vi "test json edit get or create.vi"(8 "error in (no error)":errorcluster, 11 "Enum":T1(ring)) -> (0 "error out":errorcluster, 1 "JSON out":string, 2 "JSON in":string, 3 "Passed?":bool, 5 "Result":variant)   [LabVIEW 2019, in "labview_json_tests.lvlib"]
uses:
  labview_json_tests.lvlib
  lib/JSON Action.ctl
  854176ce-6913-4507-93ff-74259bbcc79a.vi
  4f657437-8172-4485-bc80-fe3c0f5e02e5.vi
  2eb5ac62-37b8-4a64-bad4-7b844d5cb3ee.vi
  307da32d-3aea-47fb-96ba-a5907bc97348.vi
  17f0fd0c-bcdb-46ee-a433-9aeb7f125615.vi
  96cf0fb6-3c72-4f7d-8904-892807d0a1bb.vi
  59fe4560-8ba1-43eb-ba63-91e62b08ff74.vi
  8ab200a7-ddd1-4c83-9075-6b27156b72a0.vi
  151b51b3-cdff-4f44-b7cf-512c7068f231.vi
  7cf8fa0e-ed30-4591-b618-8510e1b9c6c3.vi
  7fccd278-8607-40f6-9c54-4bdcd723457c.vi
  a2037092-296c-49a0-9406-5a55253d1be9.vi
  64e50d63-3ad6-4fd6-91cf-c341bd7fd43a.vi
  fa781a07-13da-444d-a30b-150b25a8167d.vi
  8b378d6a-7cd8-4d1e-b81a-8e5d845b982b.vi
  e866194e-8ad0-44ef-85b8-025b4f165f38.vi
  ceddfd64-2eb1-41b3-96b1-c2e3a97af537.vi
  42733630-5547-4c55-90bb-661a318f8b3d.vi
  47a0a158-d444-46f2-b9cb-3651ab4d53f4.vi
  e1f56349-deab-4c5b-a68e-11cb9e1278a6.vi
  lib/JSON Edit.vi
  lib/labview_json.lvlib
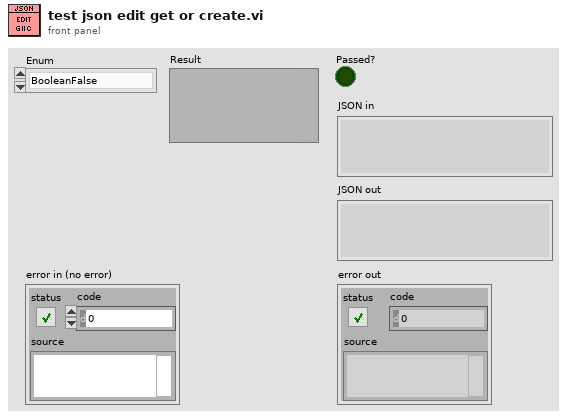
[diagram p1: front panel]
types:
  T1 = enum16{"BooleanFalse", "BooleanTrue", "StringSentence", "StringMultiline", "StringQuoted", "StringEscaped", "IntNumber", "IntMin", "IntMax", "IntI64", "IntI32", "IntI16", "IntI8", "UintNumber", "UintMin", "UintMax", "UintU64", "UintU32", "UintU16", "UintU8", "FloatNumber", "FloatMin", "FloatMax", "FloatZero", "FloatNaN", "FloatExt", "FloatDbl", "FloatSgl", "EnumU32", "EnumU16", "EnumU8", "EnumU32String", "EnumU16String", "EnumU8String", "EnumBadString", "PathAbs", "PathRel", "PathNetwork", "PathFile", "PathEmpty", "PathNaN", "PathCurrentDir", "PathParentDir", "TimeDateTime", "TimeDate", "NullVoid", "NullLVVariant", "NullBoolean", "NullInt", "NullUint", "NullFloat", "NullString", "NullPath", "NullEnum", "NullTime", "NullArray", "NullArrayVoid", "NullArrayLVVariant", "NullObject", "NullObjectVoid", "NullObjectLVVariant", "NullWaveform", "Array1DValues", "Array1DEmpty", "Array1DObject", "Array1DMulti", "Array2DValues", "Array2DEmpty", "Array3DValues", "Array3DEmpty", "ObjectValues", "ObjectEmpty", "ObjectWaveform", "ObjectReorder"}
  T2 = typedef "labview_json.lvlib/JSON Action.ctl" = enum8{"Get or Create", "Get", "Set"}
  T3 = cluster{"I16":i16, "Bool":bool, "String":string, "Array":u32[]}
  T4 = enum16{"Item A", "Item B", "Item C", "Item D", "Item E"}
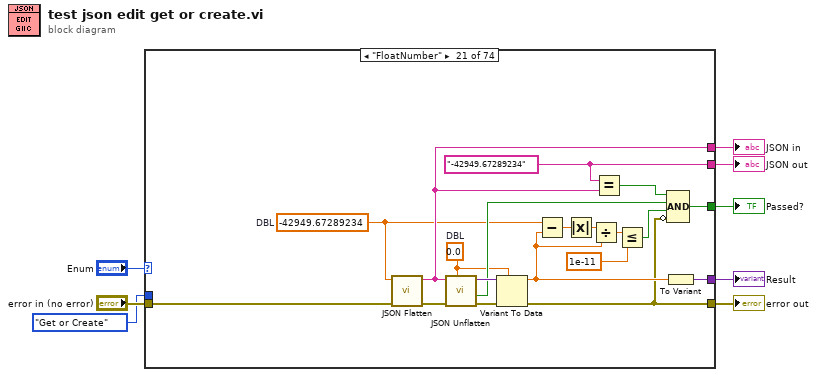
[diagram p0: block diagram]
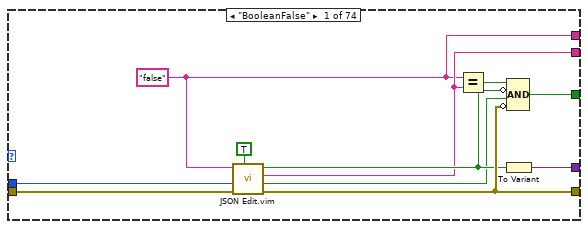
[diagram p2: hidden frame]
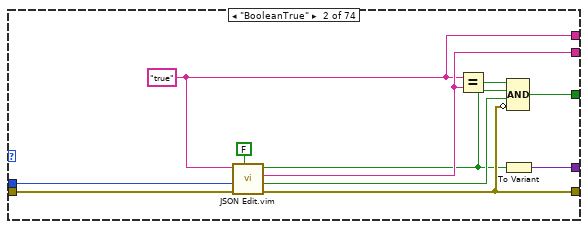
[diagram p3: hidden frame]
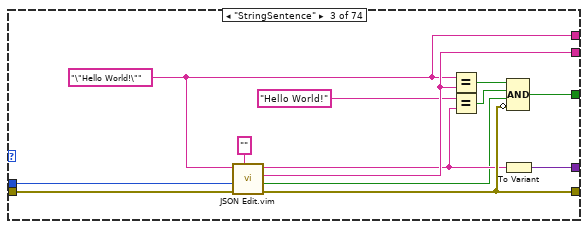
[diagram p4: hidden frame]
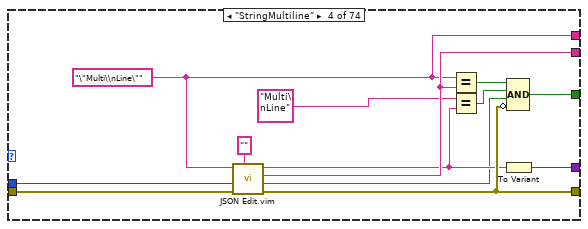
[diagram p5: hidden frame]
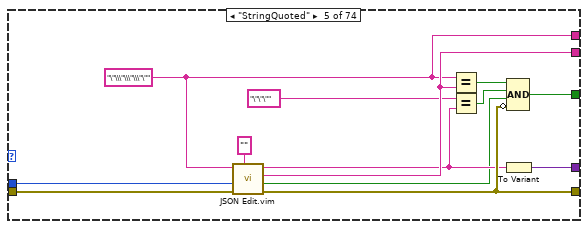
[diagram p6: hidden frame]
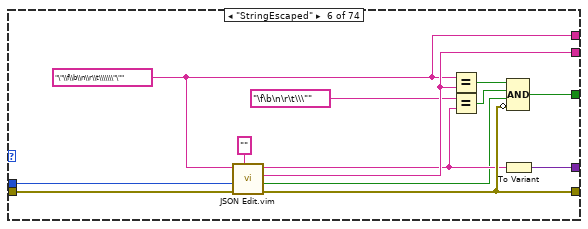
[diagram p7: hidden frame]
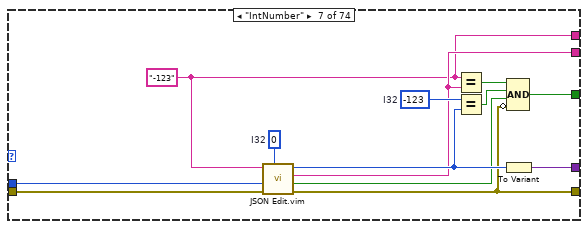
[diagram p8: hidden frame]
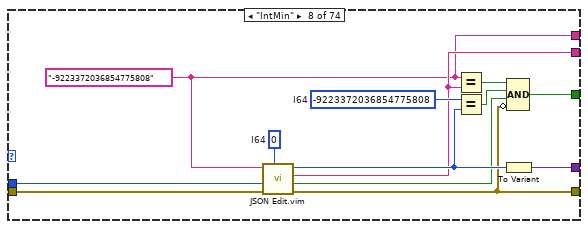
[diagram p9: hidden frame]
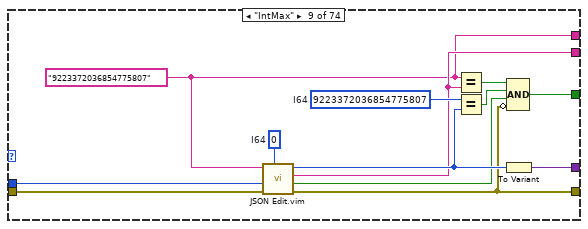
[diagram p10: hidden frame]
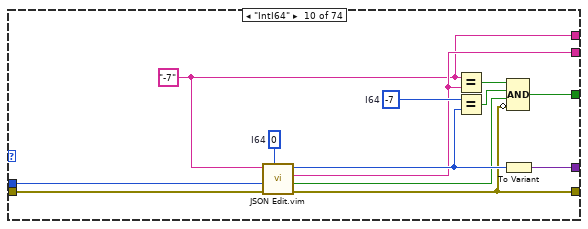
[diagram p11: hidden frame]
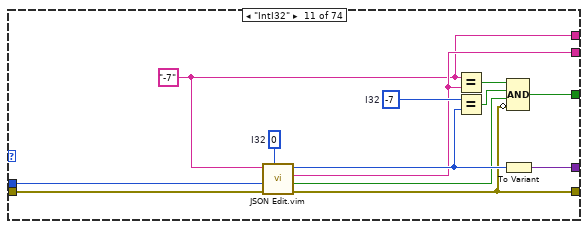
[diagram p12: hidden frame]
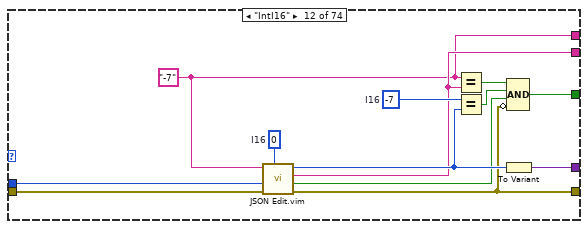
[diagram p13: hidden frame]
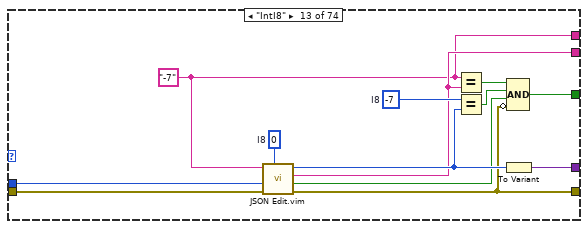
[diagram p14: hidden frame]
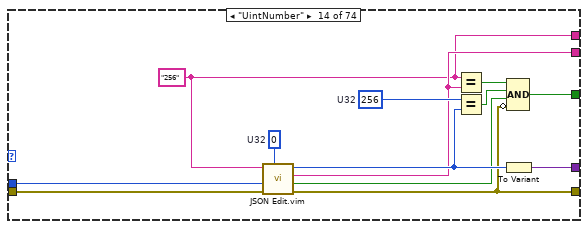
[diagram p15: hidden frame]
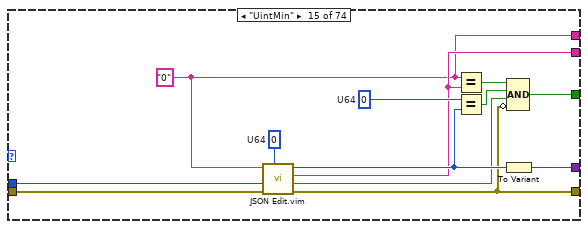
[diagram p16: hidden frame]
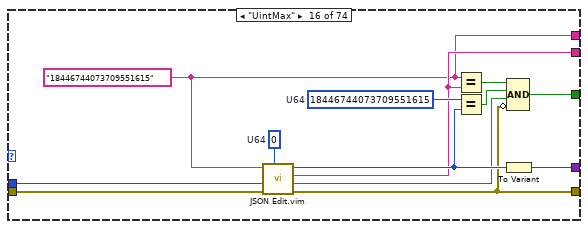
[diagram p17: hidden frame]
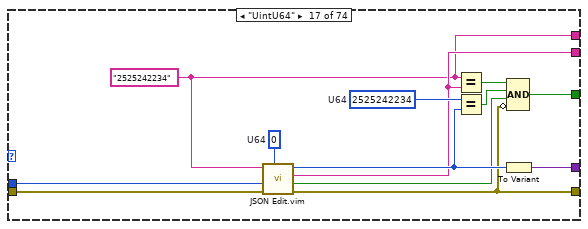
[diagram p18: hidden frame]
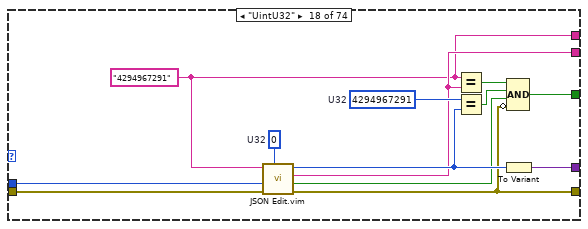
[diagram p19: hidden frame]
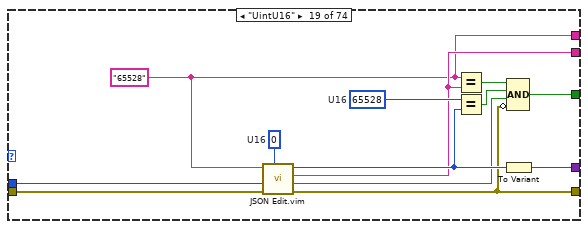
[diagram p20: hidden frame]
diagram:
  n1 = case shown="\"FloatNumber\"" "Enum" {
    tunnel: "error in (no error)" -> [w16 w27 w40 w53 w66 w79 w86 w99 w112 w125 w138 w151 w164 w177 w190 w203 w216 w229 w242 w255 w279 w294 w309 w324 w339 w358 w377 w396 w412 w428 w444 w460 w476 w492 w508 w523 w538 w553 w568 w583 w598 w613 w628 w653 w661 w690 w709 w717 w730 w743 w756 w769 w781 w794 w807 w821 w832 w846 w860 w873 w888 w901 w920 w936 w951 w983 w999 w1015 w1031 w1047 w1064 w1081 w1118 w1138]
    tunnel: [w15 w26 w39 w52 w65 w78 w89 w102 w115 w128 w141 w154 w167 w180 w193 w206 w219 w232 w245 w258 w265 w284 w299 w314 w329 w344 w363 w382 w401 w417 w433 w449 w465 w481 w498 w513 w528 w543 w558 w573 w588 w603 w618 w647 w672 w684 w699 w718 w731 w744 w757 w770 w782 w795 w808 w822 w834 w848 w861 w874 w889 w902 w910 w926 w945 w978 w989 w1005 w1021 w1037 w1058 w1075 w1115 w1132] -> w7
    tunnel: [w18 w29 w42 w55 w68 w81 w94 w107 w120 w133 w146 w159 w172 w185 w198 w211 w224 w237 w250 w263 w282 w297 w312 w327 w342 w361 w380 w399 w415 w431 w447 w463 w479 w495 w511 w526 w541 w556 w571 w586 w601 w616 w631 w656 w678 w693 w712 w723 w736 w749 w762 w775 w787 w800 w813 w827 w839 w853 w866 w879 w894 w907 w923 w939 w954 w986 w1002 w1018 w1034 w1050 w1067 w1084 w1121 w1141] -> w6
    tunnel: [w17 w28 w41 w54 w67 w80 w93 w106 w119 w132 w145 w158 w171 w184 w197 w210 w223 w236 w249 w262 w281 w296 w311 w326 w341 w360 w379 w398 w414 w430 w446 w462 w478 w494 w510 w525 w540 w555 w570 w585 w600 w615 w630 w655 w677 w692 w711 w722 w735 w748 w761 w774 w786 w799 w812 w826 w838 w852 w865 w878 w893 w906 w922 w938 w953 w985 w1001 w1017 w1033 w1049 w1066 w1083 w1120 w1140] -> w5
    tunnel: [w13 w25 w38 w51 w64 w77 w88 w101 w114 w127 w140 w153 w166 w179 w192 w205 w218 w231 w244 w257 w274 w289 w304 w319 w334 w353 w372 w391 w405 w421 w437 w453 w469 w485 w502 w516 w531 w546 w561 w576 w591 w606 w621 w635 w658 w687 w706 w714 w729 w742 w755 w768 w780 w793 w806 w820 w833 w847 w859 w872 w887 w900 w913 w929 w943 w977 w992 w1008 w1024 w1040 w1059 w1076 w1110 w1133] -> w3
    tunnel: [w12 w24 w37 w50 w63 w76 w87 w100 w113 w126 w139 w152 w165 w178 w191 w204 w217 w230 w243 w256 w277 w292 w307 w322 w337 w356 w375 w394 w410 w426 w442 w458 w474 w490 w506 w521 w536 w551 w566 w581 w596 w611 w626 w651 w658 w689 w708 w714 w729 w742 w755 w768 w780 w793 w806 w820 w833 w847 w859 w872 w887 w900 w918 w934 w949 w981 w997 w1013 w1029 w1045 w1062 w1079 w1091 w1136] -> w2
    tunnel: JSON_Action."Get or Create" ("Action (Get or Create)") -> [w10 w22 w36 w49 w62 w75 w83 w96 w109 w122 w135 w148 w161 w174 w187 w200 w213 w226 w239 w252 _ _ _ _ _ _ _ _ _ _ _ _ _ _ _ _ _ _ _ _ _ _ _ _ _ _ _ _ _ _ _ _ _ _ _ _ _ _ _ _ _ _ _ _ _ _ _ _ _ _ _ _ _ _]
    frame "BooleanFalse" {
      w12 = "false" ("JSON in")
      n2 = call "JSON Edit.vim"("Variant in"=TRUE, "error in (no error)"=w16, "Action (Get or Create)"=w10, "JSON in"=w12) -> ("error out"=w15:errorcluster, "Exists?"=w9:bool, "JSON out"=w13:string, "Variant out"=w14:bool)  [unwired: 4 in]
      n3 = Equal?(x=w12, y=w13) -> (x = y?=w19:bool)
      n4 = To Variant(anything=w14) -> (Variant=w17:variant)
      n5 = Compound Arithmetic op=AND(w19, invert w14, w9, invert w15) -> (w18:bool)
    }
    frame "BooleanTrue" {
      w24 = "true" ("JSON in")
      n6 = call "JSON Edit.vim"("Variant in"=FALSE, "error in (no error)"=w27, "Action (Get or Create)"=w22, "JSON in"=w24) -> ("error out"=w26:errorcluster, "Exists?"=w21:bool, "JSON out"=w25:string, "Variant out"=w20:bool)  [unwired: 4 in]
      n7 = Equal?(x=w24, y=w25) -> (x = y?=w30:bool)
      n8 = To Variant(anything=w20) -> (Variant=w28:variant)
      n9 = Compound Arithmetic op=AND(w30, w20, w21, invert w26) -> (w29:bool)
    }
    frame "StringSentence" {
      w37 = "\"Hello World!\"" ("JSON in")
      n10 = call "JSON Edit.vim"("Variant in"="", "error in (no error)"=w40, "Action (Get or Create)"=w36, "JSON in"=w37) -> ("error out"=w39:errorcluster, "Exists?"=w32:bool, "JSON out"=w38:string, "Variant out"=w33:string)  [unwired: 4 in]
      n11 = Equal?(x=w37, y=w38) -> (x = y?=w43:bool)
      n12 = Equal?(x="Hello World!", y=w33) -> (x = y?=w31:bool)
      n13 = To Variant(anything=w33) -> (Variant=w41:variant)
      n14 = Compound Arithmetic op=AND(w43, w31, w32, invert w39) -> (w42:bool)
    }
    frame "StringMultiline" {
      w50 = "\"Multi\\nLine\"" ("JSON in")
      n15 = call "JSON Edit.vim"("Variant in"="", "error in (no error)"=w53, "Action (Get or Create)"=w49, "JSON in"=w50) -> ("error out"=w52:errorcluster, "Exists?"=w45:bool, "JSON out"=w51:string, "Variant out"=w46:string)  [unwired: 4 in]
      n16 = Equal?(x=w50, y=w51) -> (x = y?=w56:bool)
      n17 = Equal?(x="Multi\nLine", y=w46) -> (x = y?=w44:bool)
      n18 = To Variant(anything=w46) -> (Variant=w54:variant)
      n19 = Compound Arithmetic op=AND(w56, w44, w45, invert w52) -> (w55:bool)
    }
    frame "StringQuoted" {
      w63 = "\"\\\"\\\"\\\"\"" ("JSON in")
      n20 = call "JSON Edit.vim"("Variant in"="", "error in (no error)"=w66, "Action (Get or Create)"=w62, "JSON in"=w63) -> ("error out"=w65:errorcluster, "Exists?"=w58:bool, "JSON out"=w64:string, "Variant out"=w59:string)  [unwired: 4 in]
      n21 = Equal?(x=w63, y=w64) -> (x = y?=w69:bool)
      n22 = Equal?(x="\"\"\"", y=w59) -> (x = y?=w57:bool)
      n23 = To Variant(anything=w59) -> (Variant=w67:variant)
      n24 = Compound Arithmetic op=AND(w69, w57, w58, invert w65) -> (w68:bool)
    }
    frame "StringEscaped" {
      w76 = "\"\\f\\b\\n\\r\\t\\\\\\\"\"" ("JSON in")
      n25 = call "JSON Edit.vim"("Variant in"="", "error in (no error)"=w79, "Action (Get or Create)"=w75, "JSON in"=w76) -> ("error out"=w78:errorcluster, "Exists?"=w72:bool, "JSON out"=w77:string, "Variant out"=w73:string)  [unwired: 4 in]
      n26 = Equal?(x=w76, y=w77) -> (x = y?=w82:bool)
      n27 = Equal?(x="\f\b\n\r\t\\\"", y=w73) -> (x = y?=w71:bool)
      n28 = To Variant(anything=w73) -> (Variant=w80:variant)
      n29 = Compound Arithmetic op=AND(w82, w71, w72, invert w78) -> (w81:bool)
    }
    frame "IntNumber" {
      w91 = 0  # I32
      w92 = -123  # I32
      w87 = "-123"
      n30 = call "JSON Edit.vim"("Variant in"=w91, "error in (no error)"=w86, "Action (Get or Create)"=w83, "JSON in"=w87) -> ("error out"=w89:errorcluster, "Exists?"=w85:bool, "JSON out"=w88:string, "Variant out"=w90:i32)  [unwired: 4 in]
      n31 = Equal?(x=w87, y=w88) -> (x = y?=w95:bool)
      n32 = Equal?(x=w92, y=w90) -> (x = y?=w84:bool)
      n33 = To Variant(anything=w90) -> (Variant=w93:variant)
      n34 = Compound Arithmetic op=AND(w95, w84, w85, invert w89) -> (w94:bool)
    }
    frame "IntMin" {
      w104 = i64 0  # I64
      w105 = i64 -9223372036854775808  # I64
      w100 = "-9223372036854775808"
      n35 = call "JSON Edit.vim"("Variant in"=w104, "error in (no error)"=w99, "Action (Get or Create)"=w96, "JSON in"=w100) -> ("error out"=w102:errorcluster, "Exists?"=w98:bool, "JSON out"=w101:string, "Variant out"=w103:i64)  [unwired: 4 in]
      n36 = Equal?(x=w100, y=w101) -> (x = y?=w108:bool)
      n37 = Equal?(x=w105, y=w103) -> (x = y?=w97:bool)
      n38 = To Variant(anything=w103) -> (Variant=w106:variant)
      n39 = Compound Arithmetic op=AND(w108, w97, w98, invert w102) -> (w107:bool)
    }
    frame "IntMax" {
      w117 = i64 0  # I64
      w118 = i64 9223372036854775807  # I64
      w113 = "9223372036854775807"
      n40 = call "JSON Edit.vim"("Variant in"=w117, "error in (no error)"=w112, "Action (Get or Create)"=w109, "JSON in"=w113) -> ("error out"=w115:errorcluster, "Exists?"=w111:bool, "JSON out"=w114:string, "Variant out"=w116:i64)  [unwired: 4 in]
      n41 = Equal?(x=w113, y=w114) -> (x = y?=w121:bool)
      n42 = Equal?(x=w118, y=w116) -> (x = y?=w110:bool)
      n43 = To Variant(anything=w116) -> (Variant=w119:variant)
      n44 = Compound Arithmetic op=AND(w121, w110, w111, invert w115) -> (w120:bool)
    }
    frame "IntI64" {
      w130 = i64 0  # I64
      w131 = i64 -7  # I64
      w126 = "-7"
      n45 = call "JSON Edit.vim"("Variant in"=w130, "error in (no error)"=w125, "Action (Get or Create)"=w122, "JSON in"=w126) -> ("error out"=w128:errorcluster, "Exists?"=w124:bool, "JSON out"=w127:string, "Variant out"=w129:i64)  [unwired: 4 in]
      n46 = Equal?(x=w126, y=w127) -> (x = y?=w134:bool)
      n47 = Equal?(x=w131, y=w129) -> (x = y?=w123:bool)
      n48 = To Variant(anything=w129) -> (Variant=w132:variant)
      n49 = Compound Arithmetic op=AND(w134, w123, w124, invert w128) -> (w133:bool)
    }
    frame "IntI32" {
      w143 = 0  # I32
      w144 = -7  # I32
      w139 = "-7"
      n50 = call "JSON Edit.vim"("Variant in"=w143, "error in (no error)"=w138, "Action (Get or Create)"=w135, "JSON in"=w139) -> ("error out"=w141:errorcluster, "Exists?"=w137:bool, "JSON out"=w140:string, "Variant out"=w142:i32)  [unwired: 4 in]
      n51 = Equal?(x=w139, y=w140) -> (x = y?=w147:bool)
      n52 = Equal?(x=w144, y=w142) -> (x = y?=w136:bool)
      n53 = To Variant(anything=w142) -> (Variant=w145:variant)
      n54 = Compound Arithmetic op=AND(w147, w136, w137, invert w141) -> (w146:bool)
    }
    frame "IntI16" {
      w156 = i16 0  # I16
      w157 = i16 -7  # I16
      w152 = "-7"
      n55 = call "JSON Edit.vim"("Variant in"=w156, "error in (no error)"=w151, "Action (Get or Create)"=w148, "JSON in"=w152) -> ("error out"=w154:errorcluster, "Exists?"=w150:bool, "JSON out"=w153:string, "Variant out"=w155:i16)  [unwired: 4 in]
      n56 = Equal?(x=w152, y=w153) -> (x = y?=w160:bool)
      n57 = Equal?(x=w157, y=w155) -> (x = y?=w149:bool)
      n58 = To Variant(anything=w155) -> (Variant=w158:variant)
      n59 = Compound Arithmetic op=AND(w160, w149, w150, invert w154) -> (w159:bool)
    }
    frame "IntI8" {
      w169 = i8 0  # I8
      w170 = i8 -7  # I8
      w165 = "-7"
      n60 = call "JSON Edit.vim"("Variant in"=w169, "error in (no error)"=w164, "Action (Get or Create)"=w161, "JSON in"=w165) -> ("error out"=w167:errorcluster, "Exists?"=w163:bool, "JSON out"=w166:string, "Variant out"=w168:i8)  [unwired: 4 in]
      n61 = Equal?(x=w165, y=w166) -> (x = y?=w173:bool)
      n62 = Equal?(x=w170, y=w168) -> (x = y?=w162:bool)
      n63 = To Variant(anything=w168) -> (Variant=w171:variant)
      n64 = Compound Arithmetic op=AND(w173, w162, w163, invert w167) -> (w172:bool)
    }
    frame "UintNumber" {
      w182 = u32 0  # U32
      w183 = u32 256  # U32
      w178 = "256"
      n65 = call "JSON Edit.vim"("Variant in"=w182, "error in (no error)"=w177, "Action (Get or Create)"=w174, "JSON in"=w178) -> ("error out"=w180:errorcluster, "Exists?"=w176:bool, "JSON out"=w179:string, "Variant out"=w181:u32)  [unwired: 4 in]
      n66 = Equal?(x=w178, y=w179) -> (x = y?=w186:bool)
      n67 = Equal?(x=w183, y=w181) -> (x = y?=w175:bool)
      n68 = To Variant(anything=w181) -> (Variant=w184:variant)
      n69 = Compound Arithmetic op=AND(w186, w175, w176, invert w180) -> (w185:bool)
    }
    frame "UintMin" {
      w195 = u64 0  # U64
      w196 = u64 0  # U64
      w191 = "0"
      n70 = call "JSON Edit.vim"("Variant in"=w195, "error in (no error)"=w190, "Action (Get or Create)"=w187, "JSON in"=w191) -> ("error out"=w193:errorcluster, "Exists?"=w189:bool, "JSON out"=w192:string, "Variant out"=w194:u64)  [unwired: 4 in]
      n71 = Equal?(x=w191, y=w192) -> (x = y?=w199:bool)
      n72 = Equal?(x=w196, y=w194) -> (x = y?=w188:bool)
      n73 = To Variant(anything=w194) -> (Variant=w197:variant)
      n74 = Compound Arithmetic op=AND(w199, w188, w189, invert w193) -> (w198:bool)
    }
    frame "UintMax" {
      w208 = u64 0  # U64
      w209 = u64 18446744073709551615  # U64
      w204 = "18446744073709551615"
      n75 = call "JSON Edit.vim"("Variant in"=w208, "error in (no error)"=w203, "Action (Get or Create)"=w200, "JSON in"=w204) -> ("error out"=w206:errorcluster, "Exists?"=w202:bool, "JSON out"=w205:string, "Variant out"=w207:u64)  [unwired: 4 in]
      n76 = Equal?(x=w204, y=w205) -> (x = y?=w212:bool)
      n77 = Equal?(x=w209, y=w207) -> (x = y?=w201:bool)
      n78 = To Variant(anything=w207) -> (Variant=w210:variant)
      n79 = Compound Arithmetic op=AND(w212, w201, w202, invert w206) -> (w211:bool)
    }
    frame "UintU64" {
      w221 = u64 0  # U64
      w222 = u64 2525242234  # U64
      w217 = "2525242234"
      n80 = call "JSON Edit.vim"("Variant in"=w221, "error in (no error)"=w216, "Action (Get or Create)"=w213, "JSON in"=w217) -> ("error out"=w219:errorcluster, "Exists?"=w215:bool, "JSON out"=w218:string, "Variant out"=w220:u64)  [unwired: 4 in]
      n81 = Equal?(x=w217, y=w218) -> (x = y?=w225:bool)
      n82 = Equal?(x=w222, y=w220) -> (x = y?=w214:bool)
      n83 = To Variant(anything=w220) -> (Variant=w223:variant)
      n84 = Compound Arithmetic op=AND(w225, w214, w215, invert w219) -> (w224:bool)
    }
    frame "UintU32" {
      w234 = u32 0  # U32
      w235 = u32 4294967291  # U32
      w230 = "4294967291"
      n85 = call "JSON Edit.vim"("Variant in"=w234, "error in (no error)"=w229, "Action (Get or Create)"=w226, "JSON in"=w230) -> ("error out"=w232:errorcluster, "Exists?"=w228:bool, "JSON out"=w231:string, "Variant out"=w233:u32)  [unwired: 4 in]
      n86 = Equal?(x=w230, y=w231) -> (x = y?=w238:bool)
      n87 = Equal?(x=w235, y=w233) -> (x = y?=w227:bool)
      n88 = To Variant(anything=w233) -> (Variant=w236:variant)
      n89 = Compound Arithmetic op=AND(w238, w227, w228, invert w232) -> (w237:bool)
    }
    frame "UintU16" {
      w247 = u16 0  # U16
      w248 = u16 65528  # U16
      w243 = "65528"
      n90 = call "JSON Edit.vim"("Variant in"=w247, "error in (no error)"=w242, "Action (Get or Create)"=w239, "JSON in"=w243) -> ("error out"=w245:errorcluster, "Exists?"=w241:bool, "JSON out"=w244:string, "Variant out"=w246:u16)  [unwired: 4 in]
      n91 = Equal?(x=w243, y=w244) -> (x = y?=w251:bool)
      n92 = Equal?(x=w248, y=w246) -> (x = y?=w240:bool)
      n93 = To Variant(anything=w246) -> (Variant=w249:variant)
      n94 = Compound Arithmetic op=AND(w251, w240, w241, invert w245) -> (w250:bool)
    }
    frame "UintU8" {
      w260 = u8 0  # U8
      w261 = u8 248  # U8
      w256 = "248"
      n95 = call "JSON Edit.vim"("Variant in"=w260, "error in (no error)"=w255, "Action (Get or Create)"=w252, "JSON in"=w256) -> ("error out"=w258:errorcluster, "Exists?"=w254:bool, "JSON out"=w257:string, "Variant out"=w259:u8)  [unwired: 4 in]
      n96 = Equal?(x=w256, y=w257) -> (x = y?=w264:bool)
      n97 = Equal?(x=w261, y=w259) -> (x = y?=w253:bool)
      n98 = To Variant(anything=w259) -> (Variant=w262:variant)
      n99 = Compound Arithmetic op=AND(w264, w253, w254, invert w258) -> (w263:bool)
    }
    frame "FloatNumber" {
      w273 = 0.0  # DBL
      w272 = -42949.67289234  # DBL
      w274 = "-42949.67289234"
      n100 = call "JSON Flatten.vi"("error in (no error)"=w279, "Variant in"=w272) -> ("error out"=w280:errorcluster, "JSON out"=w277:string)  [unwired: 8 in]
      n101 = call "JSON Unflatten.vi"("Variant Type"=w273, "error in (no error)"=w280, "JSON in"=w277) -> ("error out"=w278:errorcluster, "Exists?"=w275:bool, "Variant out"=w276:variant)  [unwired: 6 in]
      n102 = Variant To Data(error in=w278, type=w273, Variant=w276) -> (data=w269:dbl, error out=w265:errorcluster)
      n103 = Subtract(x=w272, y=w269) -> (x-y=w271:dbl)
      n104 = Absolute Value(x=w271) -> (abs(x)=w270:dbl)
      n105 = Divide(x=w270, y=w269) -> (x/y=w268:dbl)
      n106 = Equal?(x=w274, y=w277) -> (x = y?=w283:bool)
      n107 = Less Or Equal?(x=w268, y=1e-11) -> (x <= y?=w266:bool)
      n108 = To Variant(anything=w269) -> (Variant=w281:variant)
      n109 = Compound Arithmetic op=AND(w283, w275, w266, invert w265) -> (w282:bool)
    }
    frame "FloatMin" {
      w288 = 0.0  # DBL
      w287 = -inf  # DBL
      w289 = "-Infinity"
      n110 = call "JSON Flatten.vi"("error in (no error)"=w294, "Variant in"=w287) -> ("error out"=w295:errorcluster, "JSON out"=w292:string)  [unwired: 8 in]
      n111 = call "JSON Unflatten.vi"("Variant Type"=w288, "error in (no error)"=w295, "JSON in"=w292) -> ("error out"=w293:errorcluster, "Exists?"=w290:bool, "Variant out"=w291:variant)  [unwired: 6 in]
      n112 = Variant To Data(error in=w293, type=w288, Variant=w291) -> (data=w286:dbl, error out=w284:errorcluster)
      n113 = Equal?(x=w289, y=w292) -> (x = y?=w298:bool)
      n114 = Equal?(x=w287, y=w286) -> (x = y?=w285:bool)
      n115 = To Variant(anything=w286) -> (Variant=w296:variant)
      n116 = Compound Arithmetic op=AND(w298, w290, w285, invert w284) -> (w297:bool)
    }
    frame "FloatMax" {
      w303 = 0.0  # DBL
      w302 = inf  # DBL
      w304 = "Infinity"
      n117 = call "JSON Flatten.vi"("error in (no error)"=w309, "Variant in"=w302) -> ("error out"=w310:errorcluster, "JSON out"=w307:string)  [unwired: 8 in]
      n118 = call "JSON Unflatten.vi"("Variant Type"=w303, "error in (no error)"=w310, "JSON in"=w307) -> ("error out"=w308:errorcluster, "Exists?"=w305:bool, "Variant out"=w306:variant)  [unwired: 6 in]
      n119 = Variant To Data(error in=w308, type=w303, Variant=w306) -> (data=w301:dbl, error out=w299:errorcluster)
      n120 = Equal?(x=w304, y=w307) -> (x = y?=w313:bool)
      n121 = Equal?(x=w302, y=w301) -> (x = y?=w300:bool)
      n122 = To Variant(anything=w301) -> (Variant=w311:variant)
      n123 = Compound Arithmetic op=AND(w313, w305, w300, invert w299) -> (w312:bool)
    }
    frame "FloatZero" {
      w318 = 2.0  # DBL
      w317 = 0.0  # DBL
      w319 = "0"
      n124 = call "JSON Flatten.vi"("error in (no error)"=w324, "Variant in"=w317) -> ("error out"=w325:errorcluster, "JSON out"=w322:string)  [unwired: 8 in]
      n125 = call "JSON Unflatten.vi"("Variant Type"=w318, "error in (no error)"=w325, "JSON in"=w322) -> ("error out"=w323:errorcluster, "Exists?"=w320:bool, "Variant out"=w321:variant)  [unwired: 6 in]
      n126 = Variant To Data(error in=w323, type=w318, Variant=w321) -> (data=w316:dbl, error out=w314:errorcluster)
      n127 = Equal?(x=w319, y=w322) -> (x = y?=w328:bool)
      n128 = Equal?(x=w317, y=w316) -> (x = y?=w315:bool)
      n129 = To Variant(anything=w316) -> (Variant=w326:variant)
      n130 = Compound Arithmetic op=AND(w328, w320, w315, invert w314) -> (w327:bool)
    }
    frame "FloatNaN" {
      w333 = 2.0  # DBL
      w332 = nan  # DBL
      w334 = "NaN"
      n131 = call "JSON Flatten.vi"("error in (no error)"=w339, "Variant in"=w332) -> ("error out"=w340:errorcluster, "JSON out"=w337:string)  [unwired: 8 in]
      n132 = call "JSON Unflatten.vi"("Variant Type"=w333, "error in (no error)"=w340, "JSON in"=w337) -> ("error out"=w338:errorcluster, "Exists?"=w335:bool, "Variant out"=w336:variant)  [unwired: 6 in]
      n133 = Variant To Data(error in=w338, type=w333, Variant=w336) -> (data=w331:dbl, error out=w329:errorcluster)
      n134 = Not A Number/Path/Refnum?(number/path/refnum=w331) -> (NaN/Path/Refnum?=w330:bool)
      n135 = Equal?(x=w334, y=w337) -> (x = y?=w343:bool)
      n136 = To Variant(anything=w331) -> (Variant=w341:variant)
      n137 = Compound Arithmetic op=AND(w343, w335, w330, invert w329) -> (w342:bool)
    }
    frame "FloatExt" {
      w346 = ext 1e-13  # EXT
      w352 = ext 0.0  # EXT
      w351 = ext 1.844674407371e+19  # EXT
      w353 = "1.844674407371E+19"
      n138 = call "JSON Flatten.vi"("error in (no error)"=w358, "Variant in"=w351) -> ("error out"=w359:errorcluster, "JSON out"=w356:string)  [unwired: 8 in]
      n139 = call "JSON Unflatten.vi"("Variant Type"=w352, "error in (no error)"=w359, "JSON in"=w356) -> ("error out"=w357:errorcluster, "Exists?"=w354:bool, "Variant out"=w355:variant)  [unwired: 6 in]
      n140 = Variant To Data(error in=w357, type=w352, Variant=w355) -> (data=w348:ext, error out=w344:errorcluster)
      n141 = Subtract(x=w351, y=w348) -> (x-y=w350:ext)
      n142 = Absolute Value(x=w350) -> (abs(x)=w349:ext)
      n143 = Divide(x=w349, y=w348) -> (x/y=w347:ext)
      n144 = Equal?(x=w353, y=w356) -> (x = y?=w362:bool)
      n145 = Less Or Equal?(x=w347, y=w346) -> (x <= y?=w345:bool)
      n146 = To Variant(anything=w348) -> (Variant=w360:variant)
      n147 = Compound Arithmetic op=AND(w362, w354, w345, invert w344) -> (w361:bool)
    }
    frame "FloatDbl" {
      w365 = 1e-11  # DBL
      w371 = 0.0  # DBL
      w370 = -19273791.23844  # DBL
      w372 = "-19273791.2384399995"
      n148 = call "JSON Flatten.vi"("error in (no error)"=w377, "Variant in"=w370) -> ("error out"=w378:errorcluster, "JSON out"=w375:string)  [unwired: 8 in]
      n149 = call "JSON Unflatten.vi"("Variant Type"=w371, "error in (no error)"=w378, "JSON in"=w375) -> ("error out"=w376:errorcluster, "Exists?"=w373:bool, "Variant out"=w374:variant)  [unwired: 6 in]
      n150 = Variant To Data(error in=w376, type=w371, Variant=w374) -> (data=w367:dbl, error out=w363:errorcluster)
      n151 = Subtract(x=w370, y=w367) -> (x-y=w369:dbl)
      n152 = Absolute Value(x=w369) -> (abs(x)=w368:dbl)
      n153 = Divide(x=w368, y=w367) -> (x/y=w366:dbl)
      n154 = Equal?(x=w372, y=w375) -> (x = y?=w381:bool)
      n155 = Less Or Equal?(x=w366, y=w365) -> (x <= y?=w364:bool)
      n156 = To Variant(anything=w367) -> (Variant=w379:variant)
      n157 = Compound Arithmetic op=AND(w381, w373, w364, invert w363) -> (w380:bool)
    }
    frame "FloatSgl" {
      w384 = sgl 1e-05  # SGL
      w390 = sgl 0.0  # SGL
      w389 = sgl 82833.23  # SGL
      w391 = "82833.2265625"
      n158 = call "JSON Flatten.vi"("error in (no error)"=w396, "Variant in"=w389) -> ("error out"=w397:errorcluster, "JSON out"=w394:string)  [unwired: 8 in]
      n159 = call "JSON Unflatten.vi"("Variant Type"=w390, "error in (no error)"=w397, "JSON in"=w394) -> ("error out"=w395:errorcluster, "Exists?"=w392:bool, "Variant out"=w393:variant)  [unwired: 6 in]
      n160 = Variant To Data(error in=w395, type=w390, Variant=w393) -> (data=w386:sgl, error out=w382:errorcluster)
      n161 = Subtract(x=w389, y=w386) -> (x-y=w388:sgl)
      n162 = Absolute Value(x=w388) -> (abs(x)=w387:sgl)
      n163 = Divide(x=w387, y=w386) -> (x/y=w385:sgl)
      n164 = Equal?(x=w391, y=w394) -> (x = y?=w400:bool)
      n165 = Less Or Equal?(x=w385, y=w384) -> (x <= y?=w383:bool)
      n166 = To Variant(anything=w386) -> (Variant=w398:variant)
      n167 = Compound Arithmetic op=AND(w400, w392, w383, invert w382) -> (w399:bool)
    }
    frame "EnumU32" {
      w403 = enum32{"Item A", "Item B", "Item C", "Item D"}."Item A"  # U32
      w404 = enum32{"Item A", "Item B", "Item C", "Item D"}."Item C"  # U32
      w405 = "2"
      n168 = call "JSON Flatten.vi"("Enums as string? (F)"=FALSE, "error in (no error)"=w412, "Variant in"=w404) -> ("error out"=w413:errorcluster, "JSON out"=w410:string)  [unwired: 7 in]
      n169 = call "JSON Unflatten.vi"("Variant Type"=w403, "error in (no error)"=w413, "JSON in"=w410) -> ("error out"=w411:errorcluster, "Exists?"=w408:bool, "Variant out"=w409:variant)  [unwired: 6 in]
      n170 = Variant To Data(error in=w411, type=w403, Variant=w409) -> (data=w407:enum32{"Item A", "Item B", "Item C", "Item D"}, error out=w401:errorcluster)
      n171 = Equal?(x=w404, y=w407) -> (x = y?=w406:bool)
      n172 = Equal?(x=w405, y=w410) -> (x = y?=w416:bool)
      n173 = To Variant(anything=w407) -> (Variant=w414:variant)
      n174 = Compound Arithmetic op=AND(w416, w408, w406, invert w401) -> (w415:bool)
    }
    frame "EnumU16" {
      w419 = enum16{"Item A", "Item B", "Item C", "Item D"}."Item A"  # U16
      w420 = enum16{"Item A", "Item B", "Item C", "Item D"}."Item B"  # U16
      w421 = "1"
      n175 = call "JSON Flatten.vi"("Enums as string? (F)"=FALSE, "error in (no error)"=w428, "Variant in"=w420) -> ("error out"=w429:errorcluster, "JSON out"=w426:string)  [unwired: 7 in]
      n176 = call "JSON Unflatten.vi"("Variant Type"=w419, "error in (no error)"=w429, "JSON in"=w426) -> ("error out"=w427:errorcluster, "Exists?"=w424:bool, "Variant out"=w425:variant)  [unwired: 6 in]
      n177 = Variant To Data(error in=w427, type=w419, Variant=w425) -> (data=w423:enum16{"Item A", "Item B", "Item C", "Item D"}, error out=w417:errorcluster)
      n178 = Equal?(x=w420, y=w423) -> (x = y?=w422:bool)
      n179 = Equal?(x=w421, y=w426) -> (x = y?=w432:bool)
      n180 = To Variant(anything=w423) -> (Variant=w430:variant)
      n181 = Compound Arithmetic op=AND(w432, w424, w422, invert w417) -> (w431:bool)
    }
    frame "EnumU8" {
      w435 = enum8{"Item A", "Item B", "Item C", "Item D"}."Item A"  # U8
      w436 = enum8{"Item A", "Item B", "Item C", "Item D"}."Item C"  # U8
      w437 = "2"
      n182 = call "JSON Flatten.vi"("Enums as string? (F)"=FALSE, "error in (no error)"=w444, "Variant in"=w436) -> ("error out"=w445:errorcluster, "JSON out"=w442:string)  [unwired: 7 in]
      n183 = call "JSON Unflatten.vi"("Variant Type"=w435, "error in (no error)"=w445, "JSON in"=w442) -> ("error out"=w443:errorcluster, "Exists?"=w440:bool, "Variant out"=w441:variant)  [unwired: 6 in]
      n184 = Variant To Data(error in=w443, type=w435, Variant=w441) -> (data=w439:enum8{"Item A", "Item B", "Item C", "Item D"}, error out=w433:errorcluster)
      n185 = Equal?(x=w436, y=w439) -> (x = y?=w438:bool)
      n186 = Equal?(x=w437, y=w442) -> (x = y?=w448:bool)
      n187 = To Variant(anything=w439) -> (Variant=w446:variant)
      n188 = Compound Arithmetic op=AND(w448, w440, w438, invert w433) -> (w447:bool)
    }
    frame "EnumU32String" {
      w451 = enum32{"Item A", "Item B", "Item C", "Item D"}."Item A"  # U32
      w452 = enum32{"Item A", "Item B", "Item C", "Item D"}."Item C"  # U32
      w453 = "\"Item C\""
      n189 = call "JSON Flatten.vi"("Enums as string? (F)"=TRUE, "error in (no error)"=w460, "Variant in"=w452) -> ("error out"=w461:errorcluster, "JSON out"=w458:string)  [unwired: 7 in]
      n190 = call "JSON Unflatten.vi"("Variant Type"=w451, "error in (no error)"=w461, "JSON in"=w458) -> ("error out"=w459:errorcluster, "Exists?"=w456:bool, "Variant out"=w457:variant)  [unwired: 6 in]
      n191 = Variant To Data(error in=w459, type=w451, Variant=w457) -> (data=w455:enum32{"Item A", "Item B", "Item C", "Item D"}, error out=w449:errorcluster)
      n192 = Equal?(x=w452, y=w455) -> (x = y?=w454:bool)
      n193 = Equal?(x=w453, y=w458) -> (x = y?=w464:bool)
      n194 = To Variant(anything=w455) -> (Variant=w462:variant)
      n195 = Compound Arithmetic op=AND(w464, w456, w454, invert w449) -> (w463:bool)
    }
    frame "EnumU16String" {
      w467 = enum16{"Item A", "Item B", "Item C", "Item D"}."Item A"  # U16
      w468 = enum16{"Item A", "Item B", "Item C", "Item D"}."Item B"  # U16
      w469 = "\"Item B\""
      n196 = call "JSON Flatten.vi"("Enums as string? (F)"=TRUE, "error in (no error)"=w476, "Variant in"=w468) -> ("error out"=w477:errorcluster, "JSON out"=w474:string)  [unwired: 7 in]
      n197 = call "JSON Unflatten.vi"("Variant Type"=w467, "error in (no error)"=w477, "JSON in"=w474) -> ("error out"=w475:errorcluster, "Exists?"=w472:bool, "Variant out"=w473:variant)  [unwired: 6 in]
      n198 = Variant To Data(error in=w475, type=w467, Variant=w473) -> (data=w471:enum16{"Item A", "Item B", "Item C", "Item D"}, error out=w465:errorcluster)
      n199 = Equal?(x=w468, y=w471) -> (x = y?=w470:bool)
      n200 = Equal?(x=w469, y=w474) -> (x = y?=w480:bool)
      n201 = To Variant(anything=w471) -> (Variant=w478:variant)
      n202 = Compound Arithmetic op=AND(w480, w472, w470, invert w465) -> (w479:bool)
    }
    frame "EnumU8String" {
      w483 = enum8{"Item A", "Item B", "Item C", "Item D"}."Item A"  # U8
      w484 = enum8{"Item A", "Item B", "Item C", "Item D"}."Item C"  # U8
      w485 = "\"Item C\""
      n203 = call "JSON Flatten.vi"("Enums as string? (F)"=TRUE, "error in (no error)"=w492, "Variant in"=w484) -> ("error out"=w493:errorcluster, "JSON out"=w490:string)  [unwired: 7 in]
      n204 = call "JSON Unflatten.vi"("Variant Type"=w483, "error in (no error)"=w493, "JSON in"=w490) -> ("error out"=w491:errorcluster, "Exists?"=w488:bool, "Variant out"=w489:variant)  [unwired: 6 in]
      n205 = Variant To Data(error in=w491, type=w483, Variant=w489) -> (data=w487:enum8{"Item A", "Item B", "Item C", "Item D"}, error out=w481:errorcluster)
      n206 = Equal?(x=w484, y=w487) -> (x = y?=w486:bool)
      n207 = Equal?(x=w485, y=w490) -> (x = y?=w496:bool)
      n208 = To Variant(anything=w487) -> (Variant=w494:variant)
      n209 = Compound Arithmetic op=AND(w496, w488, w486, invert w481) -> (w495:bool)
    }
    frame "EnumBadString" {
      w500 = enum16{"Item A", "Item B", "Item C", "Item D"}."Item A"  # U16
      w501 = T4."Item E"  # U16
      w502 = "\"Item E\""
      n210 = call "JSON Flatten.vi"("Enums as string? (F)"=TRUE, "error in (no error)"=w508, "Variant in"=w501) -> ("error out"=w509:errorcluster, "JSON out"=w506:string)  [unwired: 7 in]
      n211 = call "JSON Unflatten.vi"("Variant Type"=w500, "error in (no error)"=w509, "JSON in"=w506) -> ("error out"=w507:errorcluster, "Exists?"=w504:bool, "Variant out"=w505:variant)  [unwired: 6 in]
      n212 = Variant To Data(error in=w507, type=w500, Variant=w505) -> (data=w503:enum16{"Item A", "Item B", "Item C", "Item D"}, error out=w497:errorcluster)
      n213 = Equal?(x=w502, y=w506) -> (x = y?=w512:bool)
      n214 = To Variant(anything=w503) -> (Variant=w510:variant)
      n215 = call <vilib>:"Clear Errors.vi"("error in (no error)"=w497) -> ("error out"=w498:errorcluster)  [unwired: 5 in, 1 out]
      n216 = Compound Arithmetic op=AND(w512, invert w504, w497) -> (w511:bool)
    }
    frame "PathAbs" {
      w514 = path ""
      w515 = path "C:/"
      w516 = "\"C:\\\\\""
      n217 = call "JSON Flatten.vi"("error in (no error)"=w523, "Variant in"=w515) -> ("error out"=w524:errorcluster, "JSON out"=w521:string)  [unwired: 8 in]
      n218 = call "JSON Unflatten.vi"("Variant Type"=w514, "error in (no error)"=w524, "JSON in"=w521) -> ("error out"=w522:errorcluster, "Exists?"=w519:bool, "Variant out"=w520:variant)  [unwired: 6 in]
      n219 = Variant To Data(error in=w522, type=w514, Variant=w520) -> (data=w518:path, error out=w513:errorcluster)
      n220 = Equal?(x=w515, y=w518) -> (x = y?=w517:bool)
      n221 = Equal?(x=w516, y=w521) -> (x = y?=w527:bool)
      n222 = To Variant(anything=w518) -> (Variant=w525:variant)
      n223 = Compound Arithmetic op=AND(w527, w519, w517, invert w513) -> (w526:bool)
    }
    frame "PathRel" {
      w529 = path ""
      w530 = path "abc/def.txt"
      w531 = "\"abc\\\\def.txt\""
      n224 = call "JSON Flatten.vi"("error in (no error)"=w538, "Variant in"=w530) -> ("error out"=w539:errorcluster, "JSON out"=w536:string)  [unwired: 8 in]
      n225 = call "JSON Unflatten.vi"("Variant Type"=w529, "error in (no error)"=w539, "JSON in"=w536) -> ("error out"=w537:errorcluster, "Exists?"=w534:bool, "Variant out"=w535:variant)  [unwired: 6 in]
      n226 = Variant To Data(error in=w537, type=w529, Variant=w535) -> (data=w533:path, error out=w528:errorcluster)
      n227 = Equal?(x=w530, y=w533) -> (x = y?=w532:bool)
      n228 = Equal?(x=w531, y=w536) -> (x = y?=w542:bool)
      n229 = To Variant(anything=w533) -> (Variant=w540:variant)
      n230 = Compound Arithmetic op=AND(w542, w534, w532, invert w528) -> (w541:bool)
    }
    frame "PathNetwork" {
      w544 = path ""
      w545 = path "\\\\server\\folder"
      w546 = "\"\\\\\\\\server\\\\folder\""
      n231 = call "JSON Flatten.vi"("error in (no error)"=w553, "Variant in"=w545) -> ("error out"=w554:errorcluster, "JSON out"=w551:string)  [unwired: 8 in]
      n232 = call "JSON Unflatten.vi"("Variant Type"=w544, "error in (no error)"=w554, "JSON in"=w551) -> ("error out"=w552:errorcluster, "Exists?"=w549:bool, "Variant out"=w550:variant)  [unwired: 6 in]
      n233 = Variant To Data(error in=w552, type=w544, Variant=w550) -> (data=w548:path, error out=w543:errorcluster)
      n234 = Equal?(x=w545, y=w548) -> (x = y?=w547:bool)
      n235 = Equal?(x=w546, y=w551) -> (x = y?=w557:bool)
      n236 = To Variant(anything=w548) -> (Variant=w555:variant)
      n237 = Compound Arithmetic op=AND(w557, w549, w547, invert w543) -> (w556:bool)
    }
    frame "PathFile" {
      w559 = path ""
      w560 = path "file.txt"
      w561 = "\"file.txt\""
      n238 = call "JSON Flatten.vi"("error in (no error)"=w568, "Variant in"=w560) -> ("error out"=w569:errorcluster, "JSON out"=w566:string)  [unwired: 8 in]
      n239 = call "JSON Unflatten.vi"("Variant Type"=w559, "error in (no error)"=w569, "JSON in"=w566) -> ("error out"=w567:errorcluster, "Exists?"=w564:bool, "Variant out"=w565:variant)  [unwired: 6 in]
      n240 = Variant To Data(error in=w567, type=w559, Variant=w565) -> (data=w563:path, error out=w558:errorcluster)
      n241 = Equal?(x=w560, y=w563) -> (x = y?=w562:bool)
      n242 = Equal?(x=w561, y=w566) -> (x = y?=w572:bool)
      n243 = To Variant(anything=w563) -> (Variant=w570:variant)
      n244 = Compound Arithmetic op=AND(w572, w564, w562, invert w558) -> (w571:bool)
    }
    frame "PathEmpty" {
      w574 = path ""
      w575 = path ""
      w576 = "\"\""
      n245 = call "JSON Flatten.vi"("error in (no error)"=w583, "Variant in"=w574) -> ("error out"=w584:errorcluster, "JSON out"=w581:string)  [unwired: 8 in]
      n246 = call "JSON Unflatten.vi"("Variant Type"=w575, "error in (no error)"=w584, "JSON in"=w581) -> ("error out"=w582:errorcluster, "Exists?"=w579:bool, "Variant out"=w580:variant)  [unwired: 6 in]
      n247 = Variant To Data(error in=w582, type=w575, Variant=w580) -> (data=w578:path, error out=w573:errorcluster)
      n248 = Equal?(x=w574, y=w578) -> (x = y?=w577:bool)
      n249 = Equal?(x=w576, y=w581) -> (x = y?=w587:bool)
      n250 = To Variant(anything=w578) -> (Variant=w585:variant)
      n251 = Compound Arithmetic op=AND(w587, w579, w577, invert w573) -> (w586:bool)
    }
    frame "PathNaN" {
      w589 = path ""
      w590 = path ""
      w591 = "null"
      n252 = call "JSON Flatten.vi"("error in (no error)"=w598, "Variant in"=w589) -> ("error out"=w599:errorcluster, "JSON out"=w596:string)  [unwired: 8 in]
      n253 = call "JSON Unflatten.vi"("Variant Type"=w590, "error in (no error)"=w599, "JSON in"=w596) -> ("error out"=w597:errorcluster, "Exists?"=w594:bool, "Variant out"=w595:variant)  [unwired: 6 in]
      n254 = Variant To Data(error in=w597, type=w590, Variant=w595) -> (data=w593:path, error out=w588:errorcluster)
      n255 = Equal?(x=w589, y=w593) -> (x = y?=w592:bool)
      n256 = Equal?(x=w591, y=w596) -> (x = y?=w602:bool)
      n257 = To Variant(anything=w593) -> (Variant=w600:variant)
      n258 = Compound Arithmetic op=AND(w602, w594, w592, invert w588) -> (w601:bool)
    }
    frame "PathCurrentDir" {
      w604 = path ""
      w605 = path ""
      w606 = "\".\""
      n259 = call "JSON Flatten.vi"("error in (no error)"=w613, "Variant in"=w604) -> ("error out"=w614:errorcluster, "JSON out"=w611:string)  [unwired: 8 in]
      n260 = call "JSON Unflatten.vi"("Variant Type"=w605, "error in (no error)"=w614, "JSON in"=w611) -> ("error out"=w612:errorcluster, "Exists?"=w609:bool, "Variant out"=w610:variant)  [unwired: 6 in]
      n261 = Variant To Data(error in=w612, type=w605, Variant=w610) -> (data=w608:path, error out=w603:errorcluster)
      n262 = Equal?(x=w604, y=w608) -> (x = y?=w607:bool)
      n263 = Equal?(x=w606, y=w611) -> (x = y?=w617:bool)
      n264 = To Variant(anything=w608) -> (Variant=w615:variant)
      n265 = Compound Arithmetic op=AND(w617, w609, w607, invert w603) -> (w616:bool)
    }
    frame "PathParentDir" {
      w619 = path ".."
      w620 = path ""
      w621 = "\"..\""
      n266 = call "JSON Flatten.vi"("error in (no error)"=w628, "Variant in"=w619) -> ("error out"=w629:errorcluster, "JSON out"=w626:string)  [unwired: 8 in]
      n267 = call "JSON Unflatten.vi"("Variant Type"=w620, "error in (no error)"=w629, "JSON in"=w626) -> ("error out"=w627:errorcluster, "Exists?"=w624:bool, "Variant out"=w625:variant)  [unwired: 6 in]
      n268 = Variant To Data(error in=w627, type=w620, Variant=w625) -> (data=w623:path, error out=w618:errorcluster)
      n269 = Equal?(x=w619, y=w623) -> (x = y?=w622:bool)
      n270 = Equal?(x=w621, y=w626) -> (x = y?=w632:bool)
      n271 = To Variant(anything=w623) -> (Variant=w630:variant)
      n272 = Compound Arithmetic op=AND(w632, w624, w622, invert w618) -> (w631:bool)
    }
    frame "TimeDateTime" {
      w642 = ext 1e-13  # EXT
      w646 = timestamp(0 s since 1904-01-01)
      w638 = timestamp(3677191673.3029866 s since 1904-01-01) ("Time Stamp")
      # "ISO8601"
      n273 = call "JSON Flatten.vi"("error in (no error)"=w653, "Variant in"=w638) -> ("error out"=w654:errorcluster, "JSON out"=w651:string)  [unwired: 8 in]
      n274 = call "JSON Timestamp to ISO8601.vi"("To UTC? (F)"=FALSE, "Local Date Time"=w638) -> ("ISO 8601 Date Time"=w636:string)  [unwired: 9 in]
      n275 = call "JSON Unflatten.vi"("Variant Type"=w646, "error in (no error)"=w654, "JSON in"=w651) -> ("error out"=w652:errorcluster, "Exists?"=w649:bool, "Variant out"=w650:variant)  [unwired: 6 in]
      n276 = Concatenate Strings("\"" ("string"), w636, "\"" ("string")) -> (w635:string)
      n277 = Variant To Data(error in=w652, type=w646, Variant=w650) -> (data=w648:timestamp, error out=w647:errorcluster)
      n278 = To Extended Precision Float(1:w638) -> (0:w641:ext)
      n279 = To Extended Precision Float(1:w648) -> (0:w640:ext)
      n280 = Subtract(x=w641, y=w640) -> (x-y=w645:ext)
      n281 = Equal?(x=w635, y=w651) -> (x = y?=w657:bool)
      n282 = Absolute Value(x=w645) -> (abs(x)=w644:ext)
      n283 = Divide(x=w644, y=w640) -> (x/y=w643:ext)
      n284 = Less Or Equal?(x=w643, y=w642) -> (x <= y?=w639:bool)
      n285 = To Variant(anything=w648) -> (Variant=w655:variant)
      n286 = Compound Arithmetic op=AND(w657, w649, w639, invert w647) -> (w656:bool)
    }
    frame "TimeDate" {
      w659 = "2020-11-13" ("JSON in")
      w667 = ext 1e-13  # EXT
      w671 = timestamp(0 s since 1904-01-01)
      # "ISO8601"
      n287 = call "JSON ISO8601 to Timestamp.vi"("ISO 8601 Date Time"=w659) -> ("Local Time Stamp"=w660:timestamp)  [unwired: 10 in]
      n288 = Concatenate Strings("\"" ("string"), w659, "\"" ("string")) -> (w658:string)
      n289 = call "JSON Unflatten.vi"("Variant Type"=w671, "error in (no error)"=w661, "JSON in"=w658) -> ("error out"=w676:errorcluster, "Exists?"=w674:bool, "Variant out"=w675:variant)  [unwired: 6 in]
      n290 = Variant To Data(error in=w676, type=w671, Variant=w675) -> (data=w673:timestamp, error out=w672:errorcluster)
      n291 = To Extended Precision Float(1:w660) -> (0:w666:ext)
      n292 = To Extended Precision Float(1:w673) -> (0:w665:ext)
      n293 = Subtract(x=w666, y=w665) -> (x-y=w670:ext)
      n294 = Equal?(x=w658, y=w658) -> (x = y?=w679:bool)
      n295 = Absolute Value(x=w670) -> (abs(x)=w669:ext)
      n296 = Divide(x=w669, y=w665) -> (x/y=w668:ext)
      n297 = Less Or Equal?(x=w668, y=w667) -> (x <= y?=w664:bool)
      n298 = To Variant(anything=w673) -> (Variant=w677:variant)
      n299 = Compound Arithmetic op=AND(w679, w674, w664, invert w672) -> (w678:bool)
    }
    frame "NullVoid" {
      w683 = variant
      w687 = "null"
      # "Variant to Data on void\ncauses error 1"
      n300 = call "JSON Flatten.vi"("error in (no error)"=w690, "Variant in"=w683) -> ("error out"=w691:errorcluster, "JSON out"=w689:string)  [unwired: 8 in]
      n301 = call "JSON Unflatten.vi"("Variant Type"=variant, "error in (no error)"=w691, "JSON in"=w689) -> ("error out"=w684:errorcluster, "Exists?"=w688:bool, "Variant out"=w682:variant)  [unwired: 6 in]
      n302 = Variant To Flattened String(Variant=w683) -> (data string=w681:string)  [unwired: 1 out]
      n303 = Variant To Flattened String(Variant=w682) -> (data string=w680:string)  [unwired: 1 out]
      n304 = Equal?(x=w681, y=w680) -> (x = y?=w686:bool)
      n305 = Equal?(x=w687, y=w689) -> (x = y?=w694:bool)
      n306 = To Variant(anything=w682) -> (Variant=w692:variant)
      n307 = Compound Arithmetic op=AND(w694, w688, w686, invert w684) -> (w693:bool)
    }
    frame "NullLVVariant" {
      w696 = variant
      w695 = variant
      w706 = "null"
      n308 = To Variant(anything=w695) -> (Variant=w701:variant)
      n309 = call "JSON Flatten.vi"("error in (no error)"=w709, "Variant in"=w701) -> ("error out"=w710:errorcluster, "JSON out"=w708:string)  [unwired: 8 in]
      n310 = To Variant(anything=w696) -> (Variant=w700:variant)
      n311 = call "JSON Unflatten.vi"("Variant Type"=w700, "error in (no error)"=w710, "JSON in"=w708) -> ("error out"=w704:errorcluster, "Exists?"=w707:bool, "Variant out"=w698:variant)  [unwired: 6 in]
      n312 = Variant To Data(error in=w704, type=w696, Variant=w698) -> (data=w697:variant, error out=w699:errorcluster)
      n313 = Variant To Flattened String(Variant=w695) -> (data string=w703:string)  [unwired: 1 out]
      n314 = Variant To Flattened String(Variant=w697) -> (data string=w702:string)  [unwired: 1 out]
      n315 = Equal?(x=w703, y=w702) -> (x = y?=w705:bool)
      n316 = Equal?(x=w706, y=w708) -> (x = y?=w713:bool)
      n317 = To Variant(anything=w697) -> (Variant=w711:variant)
      n318 = Compound Arithmetic op=AND(w713, w707, w705, invert w699) -> (w712:bool)
    }
    frame "NullBoolean" {
      w716 = TRUE
      w714 = "null"
      n319 = call "JSON Unflatten.vi"("Variant Type"=w716, "error in (no error)"=w717, "JSON in"=w714) -> ("error out"=w721:errorcluster, "Exists?"=w719:bool, "Variant out"=w720:variant)  [unwired: 6 in]
      n320 = Variant To Data(error in=w721, type=w716, Variant=w720) -> (data=w715:bool, error out=w718:errorcluster)
      n321 = Equal?(x=w714, y=w714) -> (x = y?=w724:bool)
      n322 = To Variant(anything=w715) -> (Variant=w722:variant)
      n323 = Compound Arithmetic op=AND(w724, w719, invert w715, invert w718) -> (w723:bool)
    }
    frame "NullInt" {
      w726 = 0  # I32
      w728 = -1  # I32
      w729 = "null"
      n324 = call "JSON Unflatten.vi"("Variant Type"=w728, "error in (no error)"=w730, "JSON in"=w729) -> ("error out"=w734:errorcluster, "Exists?"=w732:bool, "Variant out"=w733:variant)  [unwired: 6 in]
      n325 = Variant To Data(error in=w734, type=w728, Variant=w733) -> (data=w727:i32, error out=w731:errorcluster)
      n326 = Equal?(x=w726, y=w727) -> (x = y?=w725:bool)
      n327 = Equal?(x=w729, y=w729) -> (x = y?=w737:bool)
      n328 = To Variant(anything=w727) -> (Variant=w735:variant)
      n329 = Compound Arithmetic op=AND(w737, w732, w725, invert w731) -> (w736:bool)
    }
    frame "NullUint" {
      w739 = u32 0  # U32
      w741 = u32 1  # U32
      w742 = "null"
      n330 = call "JSON Unflatten.vi"("Variant Type"=w741, "error in (no error)"=w743, "JSON in"=w742) -> ("error out"=w747:errorcluster, "Exists?"=w745:bool, "Variant out"=w746:variant)  [unwired: 6 in]
      n331 = Variant To Data(error in=w747, type=w741, Variant=w746) -> (data=w740:u32, error out=w744:errorcluster)
      n332 = Equal?(x=w739, y=w740) -> (x = y?=w738:bool)
      n333 = Equal?(x=w742, y=w742) -> (x = y?=w750:bool)
      n334 = To Variant(anything=w740) -> (Variant=w748:variant)
      n335 = Compound Arithmetic op=AND(w750, w745, w738, invert w744) -> (w749:bool)
    }
    frame "NullFloat" {
      w752 = 0.0  # DBL
      w754 = 1.0  # DBL
      w755 = "null"
      n336 = call "JSON Unflatten.vi"("Variant Type"=w754, "error in (no error)"=w756, "JSON in"=w755) -> ("error out"=w760:errorcluster, "Exists?"=w758:bool, "Variant out"=w759:variant)  [unwired: 6 in]
      n337 = Variant To Data(error in=w760, type=w754, Variant=w759) -> (data=w753:dbl, error out=w757:errorcluster)
      n338 = Equal?(x=w752, y=w753) -> (x = y?=w751:bool)
      n339 = Equal?(x=w755, y=w755) -> (x = y?=w763:bool)
      n340 = To Variant(anything=w753) -> (Variant=w761:variant)
      n341 = Compound Arithmetic op=AND(w763, w758, w751, invert w757) -> (w762:bool)
    }
    frame "NullString" {
      w767 = "x"
      w768 = "null"
      n342 = call "JSON Unflatten.vi"("Variant Type"=w767, "error in (no error)"=w769, "JSON in"=w768) -> ("error out"=w773:errorcluster, "Exists?"=w771:bool, "Variant out"=w772:variant)  [unwired: 6 in]
      n343 = Variant To Data(error in=w773, type=w767, Variant=w772) -> (data=w766:string, error out=w770:errorcluster)
      n344 = Equal?(x="", y=w766) -> (x = y?=w764:bool)
      n345 = Equal?(x=w768, y=w768) -> (x = y?=w776:bool)
      n346 = To Variant(anything=w766) -> (Variant=w774:variant)
      n347 = Compound Arithmetic op=AND(w776, w771, w764, invert w770) -> (w775:bool)
    }
    frame "NullPath" {
      w779 = path "C:/"
      w780 = "null"
      n348 = call "JSON Unflatten.vi"("Variant Type"=w779, "error in (no error)"=w781, "JSON in"=w780) -> ("error out"=w785:errorcluster, "Exists?"=w783:bool, "Variant out"=w784:variant)  [unwired: 6 in]
      n349 = Variant To Data(error in=w785, type=w779, Variant=w784) -> (data=w778:path, error out=w782:errorcluster)
      n350 = Not A Number/Path/Refnum?(number/path/refnum=w778) -> (NaN/Path/Refnum?=w777:bool)
      n351 = Equal?(x=w780, y=w780) -> (x = y?=w788:bool)
      n352 = To Variant(anything=w778) -> (Variant=w786:variant)
      n353 = Compound Arithmetic op=AND(w788, w783, w777, invert w782) -> (w787:bool)
    }
    frame "NullEnum" {
      w790 = enum16{"Item A", "Item B", "Item C"}."Item B"
      w793 = "null"
      n354 = call "JSON Unflatten.vi"("Variant Type"=w790, "error in (no error)"=w794, "JSON in"=w793) -> ("error out"=w798:errorcluster, "Exists?"=w796:bool, "Variant out"=w797:variant)  [unwired: 6 in]
      n355 = Variant To Data(error in=w798, type=w790, Variant=w797) -> (data=w792:enum16{"Item A", "Item B", "Item C"}, error out=w795:errorcluster)
      n356 = Equal?(x=enum16{"Item A", "Item B", "Item C"}."Item A", y=w792) -> (x = y?=w791:bool)
      n357 = Equal?(x=w793, y=w793) -> (x = y?=w801:bool)
      n358 = To Variant(anything=w792) -> (Variant=w799:variant)
      n359 = Compound Arithmetic op=AND(w801, w796, w791, invert w795) -> (w800:bool)
    }
    frame "NullTime" {
      w803 = timestamp(3688247390.302975 s since 1904-01-01) ("Time Stamp")
      w806 = "null"
      n360 = call "JSON Unflatten.vi"("Variant Type"=w803, "error in (no error)"=w807, "JSON in"=w806) -> ("error out"=w811:errorcluster, "Exists?"=w809:bool, "Variant out"=w810:variant)  [unwired: 6 in]
      n361 = Variant To Data(error in=w811, type=w803, Variant=w810) -> (data=w805:timestamp, error out=w808:errorcluster)
      n362 = Equal?(x=timestamp(0 s since 1904-01-01), y=w805) -> (x = y?=w804:bool)
      n363 = Equal?(x=w806, y=w806) -> (x = y?=w814:bool)
      n364 = To Variant(anything=w805) -> (Variant=w812:variant)
      n365 = Compound Arithmetic op=AND(w814, w809, w804, invert w808) -> (w813:bool)
    }
    frame "NullArray" {
      w817 = string[] ["a"]
      w820 = "null"
      n366 = call "JSON Unflatten.vi"("Variant Type"=w817, "error in (no error)"=w821, "JSON in"=w820) -> ("error out"=w825:errorcluster, "Exists?"=w823:bool, "Variant out"=w824:variant)  [unwired: 6 in]
      n367 = Variant To Data(error in=w825, type=w817, Variant=w824) -> (data=w819:string[], error out=w822:errorcluster)
      n368 = Equal?(x=string[] [], y=w819) -> (x = y?=w818:bool[])
      n369 = And Array Elements(Boolean array=w818) -> (logical AND=w815:bool)
      n370 = Equal?(x=w820, y=w820) -> (x = y?=w828:bool)
      n371 = To Variant(anything=w819) -> (Variant=w826:variant)
      n372 = Compound Arithmetic op=AND(w828, w823, w815, invert w822) -> (w827:bool)
    }
    frame "NullArrayVoid" {
      w831 = variant[] []
      w833 = "null"
      n373 = call "JSON Unflatten.vi"("Variant Type"=w831, "error in (no error)"=w832, "JSON in"=w833) -> ("error out"=w837:errorcluster, "Exists?"=w835:bool, "Variant out"=w836:variant)  [unwired: 6 in]
      n374 = Variant To Data(error in=w837, type=w831, Variant=w836) -> (data=w830:variant[], error out=w834:errorcluster)
      n375 = Empty Array?(array=w830) -> (empty?=w829:bool)
      n376 = Equal?(x=w833, y=w833) -> (x = y?=w840:bool)
      n377 = To Variant(anything=w830) -> (Variant=w838:variant)
      n378 = Compound Arithmetic op=AND(w840, w835, w829, invert w834) -> (w839:bool)
    }
    frame "NullArrayLVVariant" {
      w847 = "null"
      n379 = To Variant(anything=variant) -> (Variant=w842:variant)
      n380 = Build Array(w842) -> (w841:variant[])
      n381 = call "JSON Unflatten.vi"("Variant Type"=w841, "error in (no error)"=w846, "JSON in"=w847) -> ("error out"=w851:errorcluster, "Exists?"=w849:bool, "Variant out"=w850:variant)  [unwired: 6 in]
      n382 = Variant To Data(error in=w851, type=w841, Variant=w850) -> (data=w845:variant[], error out=w848:errorcluster)
      n383 = Empty Array?(array=w845) -> (empty?=w844:bool)
      n384 = Equal?(x=w847, y=w847) -> (x = y?=w854:bool)
      n385 = To Variant(anything=w845) -> (Variant=w852:variant)
      n386 = Compound Arithmetic op=AND(w854, w849, w844, invert w848) -> (w853:bool)
    }
    frame "NullObject" {
      w857 = T3 {"I16"=1, "Bool"=TRUE, "String"="a", "Array"=[1]} ("Cluster")
      w859 = "null"
      n387 = call "JSON Unflatten.vi"("Variant Type"=w857, "error in (no error)"=w860, "JSON in"=w859) -> ("error out"=w864:errorcluster, "Exists?"=w862:bool, "Variant out"=w863:variant)  [unwired: 6 in]
      n388 = Variant To Data(error in=w864, type=w857, Variant=w863) -> (data=w858:T3, error out=w861:errorcluster)
      n389 = Equal?(x=T3 {"I16"=0, "Bool"=FALSE, "String"="", "Array"=[]} ("Cluster"), y=w858) -> (x = y?=w855:bool)
      n390 = Equal?(x=w859, y=w859) -> (x = y?=w867:bool)
      n391 = To Variant(anything=w858) -> (Variant=w865:variant)
      n392 = Compound Arithmetic op=AND(w867, w862, w855, invert w861) -> (w866:bool)
    }
    frame "NullObjectVoid" {
      w869 = cluster{variant} {variant}
      w872 = "null"
      n393 = call "JSON Unflatten.vi"("Variant Type"=w869, "error in (no error)"=w873, "JSON in"=w872) -> ("error out"=w877:errorcluster, "Exists?"=w875:bool, "Variant out"=w876:variant)  [unwired: 6 in]
      n394 = Variant To Data(error in=w877, type=w869, Variant=w876) -> (data=w871:cluster{variant}, error out=w874:errorcluster)
      n395 = Equal?(x=cluster{variant} {variant}, y=w871) -> (x = y?=w870:bool)
      n396 = Equal?(x=w872, y=w872) -> (x = y?=w880:bool)
      n397 = To Variant(anything=w871) -> (Variant=w878:variant)
      n398 = Compound Arithmetic op=AND(w880, w875, w870, invert w874) -> (w879:bool)
    }
    frame "NullObjectLVVariant" {
      w882 = variant
      w887 = "null"
      n399 = To Variant(anything=w882) -> (Variant=w885:variant)
      n400 = Bundle("Variant"=w885) -> (w884:cluster{"Variant":variant})  [unwired: 1 in]
      n401 = call "JSON Unflatten.vi"("Variant Type"=w884, "error in (no error)"=w888, "JSON in"=w887) -> ("error out"=w892:errorcluster, "Exists?"=w890:bool, "Variant out"=w891:variant)  [unwired: 6 in]
      n402 = Variant To Data(error in=w892, type=w884, Variant=w891) -> (data=w883:cluster{"Variant":variant}, error out=w889:errorcluster)
      n403 = Unbundle By Name(w883) -> ("Variant"=w881:variant)
      n404 = Equal?(x=w882, y=w881) -> (x = y?=w886:bool)
      n405 = Equal?(x=w887, y=w887) -> (x = y?=w895:bool)
      n406 = To Variant(anything=w883) -> (Variant=w893:variant)
      n407 = Compound Arithmetic op=AND(w895, w890, w886, invert w889) -> (w894:bool)
    }
    frame "NullWaveform" {
      w897 = waveform(dbl) {"t0"=timestamp(3681289404.123456 s since 1904-01-01), "dt"=0.5, "Y"=[1.1, 2.2, 3.3]} ("Waveform")
      w900 = "null"
      n408 = call "JSON Unflatten.vi"("Variant Type"=w897, "error in (no error)"=w901, "JSON in"=w900) -> ("error out"=w905:errorcluster, "Exists?"=w903:bool, "Variant out"=w904:variant)  [unwired: 6 in]
      n409 = Variant To Data(error in=w905, type=w897, Variant=w904) -> (data=w899:waveform(dbl), error out=w902:errorcluster)
      n410 = Equal?(x=waveform(dbl) {"t0"=timestamp(0 s since 1904-01-01), "dt"=0.0, "Y"=[]} ("Waveform"), y=w899) -> (x = y?=w898:bool)
      n411 = Equal?(x=w900, y=w900) -> (x = y?=w908:bool)
      n412 = To Variant(anything=w899) -> (Variant=w906:variant)
      n413 = Compound Arithmetic op=AND(w908, w903, w898, invert w902) -> (w907:bool)
    }
    frame "Array1DValues" {
      w911 = i32[] []  # I32
      w912 = i32[] [1, 2, 3]  # I32
      w913 = "[1,2,3]"
      n414 = call "JSON Flatten.vi"("error in (no error)"=w920, "Variant in"=w912) -> ("error out"=w921:errorcluster, "JSON out"=w918:string)  [unwired: 8 in]
      n415 = call "JSON Unflatten.vi"("Variant Type"=w911, "error in (no error)"=w921, "JSON in"=w918) -> ("error out"=w919:errorcluster, "Exists?"=w916:bool, "Variant out"=w917:variant)  [unwired: 6 in]
      n416 = Variant To Data(error in=w919, type=w911, Variant=w917) -> (data=w915:i32[], error out=w910:errorcluster)
      n417 = Equal?(x=w912, y=w915) -> (x = y?=w914:bool[])
      n418 = And Array Elements(Boolean array=w914) -> (logical AND=w909:bool)
      n419 = Equal?(x=w913, y=w918) -> (x = y?=w924:bool)
      n420 = To Variant(anything=w915) -> (Variant=w922:variant)
      n421 = Compound Arithmetic op=AND(w924, w916, w909, invert w910) -> (w923:bool)
    }
    frame "Array1DEmpty" {
      w927 = i32[] [1]  # I32
      w928 = i32[] []  # I32
      w929 = "[]"
      n422 = call "JSON Flatten.vi"("error in (no error)"=w936, "Variant in"=w928) -> ("error out"=w937:errorcluster, "JSON out"=w934:string)  [unwired: 8 in]
      n423 = call "JSON Unflatten.vi"("Variant Type"=w927, "error in (no error)"=w937, "JSON in"=w934) -> ("error out"=w935:errorcluster, "Exists?"=w932:bool, "Variant out"=w933:variant)  [unwired: 6 in]
      n424 = Variant To Data(error in=w935, type=w927, Variant=w933) -> (data=w931:i32[], error out=w926:errorcluster)
      n425 = Equal?(x=w928, y=w931) -> (x = y?=w930:bool[])
      n426 = And Array Elements(Boolean array=w930) -> (logical AND=w925:bool)
      n427 = Equal?(x=w929, y=w934) -> (x = y?=w940:bool)
      n428 = To Variant(anything=w931) -> (Variant=w938:variant)
      n429 = Compound Arithmetic op=AND(w940, w932, w925, invert w926) -> (w939:bool)
    }
    frame "Array1DObject" {
      w942 = errorcluster[] []
      w943 = "[{\"status\":true,\"code\":8,\"source\":\"abc\"},{\"status\":false,\"code\":9,\"source\":\"def\"},{\"status\":true,\"code\":10,\"source\":\"ghi\"}]"
      w944 = errorcluster[] [{"status"=TRUE, "code"=8, "source"="abc"}, {"status"=FALSE, "code"=9, "source"="def"}, {"status"=TRUE, "code"=10, "source"="ghi"}]
      n430 = call "JSON Flatten.vi"("error in (no error)"=w951, "Variant in"=w944) -> ("error out"=w952:errorcluster, "JSON out"=w949:string)  [unwired: 8 in]
      n431 = call "JSON Unflatten.vi"("Variant Type"=w942, "error in (no error)"=w952, "JSON in"=w949) -> ("error out"=w950:errorcluster, "Exists?"=w947:bool, "Variant out"=w948:variant)  [unwired: 6 in]
      n432 = Variant To Data(error in=w950, type=w942, Variant=w948) -> (data=w946:errorcluster[], error out=w945:errorcluster)
      n433 = Equal?(x=w944, y=w946) -> (x = y?=w941:bool)
      n434 = Equal?(x=w943, y=w949) -> (x = y?=w955:bool)
      n435 = To Variant(anything=w946) -> (Variant=w953:variant)
      n436 = Compound Arithmetic op=AND(w955, w947, w941, invert w945) -> (w954:bool)
    }
    frame "Array1DMulti" {
      w977 = "[true,3,\"abc\",{\"status\":true,\"code\":10,\"source\":\"ghi\"}]"
      # "Note: Multityped array data must be built into the variant array\nso that the variant type definitions can parse the data successfully"
      n437 = To Variant(anything=FALSE) -> (Variant=w961:variant)
      n438 = To Variant(anything=u64 0) -> (Variant=w963:variant)
      n439 = To Variant(anything="") -> (Variant=w965:variant)
      n440 = To Variant(anything=errorcluster {"status"=FALSE, "code"=0, "source"=""} ("error out")) -> (Variant=w967:variant)
      n441 = To Variant(anything=TRUE) -> (Variant=w975:variant)
      n442 = To Variant(anything=u64 3) -> (Variant=w973:variant)
      n443 = To Variant(anything="abc") -> (Variant=w971:variant)
      n444 = To Variant(anything=errorcluster {"status"=TRUE, "code"=10, "source"="ghi"} ("error out")) -> (Variant=w969:variant)
      n445 = Build Array(w961, w963, w965, w967) -> (w959:variant[])
      n446 = Build Array(w975, w973, w971, w969) -> (w958:variant[])
      n447 = call "JSON Flatten.vi"("error in (no error)"=w983, "Variant in"=w958) -> ("error out"=w984:errorcluster, "JSON out"=w981:string)  [unwired: 8 in]
      n448 = call "JSON Unflatten.vi"("Variant Type"=w959, "error in (no error)"=w984, "JSON in"=w981) -> ("error out"=w982:errorcluster, "Exists?"=w979:bool, "Variant out"=w980:variant)  [unwired: 6 in]
      n449 = Variant To Data(error in=w982, type=w959, Variant=w980) -> (data=w957:variant[], error out=w978:errorcluster)
      n450 = Equal?(x=w958, y=w957) -> (x = y?=w956:bool[])
      n451 = Equal?(x=w977, y=w981) -> (x = y?=w987:bool)
      n452 = And Array Elements(Boolean array=w956) -> (logical AND=w968:bool)
      n453 = To Variant(anything=w957) -> (Variant=w985:variant)
      n454 = Compound Arithmetic op=AND(w987, w979, w968, invert w978) -> (w986:bool)
    }
    frame "Array2DValues" {
      w990 = i32[][] []  # I32
      w991 = i32[][] [[1, 2, 3], [4, 5, 6]]  # I32
      w992 = "[[1,2,3],[4,5,6]]"
      n455 = call "JSON Flatten.vi"("error in (no error)"=w999, "Variant in"=w991) -> ("error out"=w1000:errorcluster, "JSON out"=w997:string)  [unwired: 8 in]
      n456 = call "JSON Unflatten.vi"("Variant Type"=w990, "error in (no error)"=w1000, "JSON in"=w997) -> ("error out"=w998:errorcluster, "Exists?"=w995:bool, "Variant out"=w996:variant)  [unwired: 6 in]
      n457 = Variant To Data(error in=w998, type=w990, Variant=w996) -> (data=w994:i32[][], error out=w989:errorcluster)
      n458 = Equal?(x=w991, y=w994) -> (x = y?=w993:bool[][])
      n459 = And Array Elements(Boolean array=w993) -> (logical AND=w988:bool)
      n460 = Equal?(x=w992, y=w997) -> (x = y?=w1003:bool)
      n461 = To Variant(anything=w994) -> (Variant=w1001:variant)
      n462 = Compound Arithmetic op=AND(w1003, w995, w988, invert w989) -> (w1002:bool)
    }
    frame "Array2DEmpty" {
      w1006 = i32[][] [[1]]  # I32
      w1007 = i32[][] []  # I32
      w1008 = "[]"
      n463 = call "JSON Flatten.vi"("error in (no error)"=w1015, "Variant in"=w1007) -> ("error out"=w1016:errorcluster, "JSON out"=w1013:string)  [unwired: 8 in]
      n464 = call "JSON Unflatten.vi"("Variant Type"=w1006, "error in (no error)"=w1016, "JSON in"=w1013) -> ("error out"=w1014:errorcluster, "Exists?"=w1011:bool, "Variant out"=w1012:variant)  [unwired: 6 in]
      n465 = Variant To Data(error in=w1014, type=w1006, Variant=w1012) -> (data=w1010:i32[][], error out=w1005:errorcluster)
      n466 = Equal?(x=w1007, y=w1010) -> (x = y?=w1009:bool[][])
      n467 = And Array Elements(Boolean array=w1009) -> (logical AND=w1004:bool)
      n468 = Equal?(x=w1008, y=w1013) -> (x = y?=w1019:bool)
      n469 = To Variant(anything=w1010) -> (Variant=w1017:variant)
      n470 = Compound Arithmetic op=AND(w1019, w1011, w1004, invert w1005) -> (w1018:bool)
    }
    frame "Array3DValues" {
      w1022 = i32[][][] []  # I32
      w1023 = i32[][][] [[[1, 2, 3], [4, 5, 6]], [[7, 8, 0], [0, 0, 9]]]  # I32
      w1024 = "[[[1,2,3],[4,5,6]],[[7,8,0],[0,0,9]]]"
      n471 = call "JSON Flatten.vi"("error in (no error)"=w1031, "Variant in"=w1023) -> ("error out"=w1032:errorcluster, "JSON out"=w1029:string)  [unwired: 8 in]
      n472 = call "JSON Unflatten.vi"("Variant Type"=w1022, "error in (no error)"=w1032, "JSON in"=w1029) -> ("error out"=w1030:errorcluster, "Exists?"=w1027:bool, "Variant out"=w1028:variant)  [unwired: 6 in]
      n473 = Variant To Data(error in=w1030, type=w1022, Variant=w1028) -> (data=w1026:i32[][][], error out=w1021:errorcluster)
      n474 = Equal?(x=w1023, y=w1026) -> (x = y?=w1025:bool[][][])
      n475 = And Array Elements(Boolean array=w1025) -> (logical AND=w1020:bool)
      n476 = Equal?(x=w1024, y=w1029) -> (x = y?=w1035:bool)
      n477 = To Variant(anything=w1026) -> (Variant=w1033:variant)
      n478 = Compound Arithmetic op=AND(w1035, w1027, w1020, invert w1021) -> (w1034:bool)
    }
    frame "Array3DEmpty" {
      w1038 = i32[][][] [[[1]]]  # I32
      w1039 = i32[][][] []  # I32
      w1040 = "[]"
      n479 = call "JSON Flatten.vi"("error in (no error)"=w1047, "Variant in"=w1039) -> ("error out"=w1048:errorcluster, "JSON out"=w1045:string)  [unwired: 8 in]
      n480 = call "JSON Unflatten.vi"("Variant Type"=w1038, "error in (no error)"=w1048, "JSON in"=w1045) -> ("error out"=w1046:errorcluster, "Exists?"=w1043:bool, "Variant out"=w1044:variant)  [unwired: 6 in]
      n481 = Variant To Data(error in=w1046, type=w1038, Variant=w1044) -> (data=w1042:i32[][][], error out=w1037:errorcluster)
      n482 = Equal?(x=w1039, y=w1042) -> (x = y?=w1041:bool[][][])
      n483 = And Array Elements(Boolean array=w1041) -> (logical AND=w1036:bool)
      n484 = Equal?(x=w1040, y=w1045) -> (x = y?=w1051:bool)
      n485 = To Variant(anything=w1042) -> (Variant=w1049:variant)
      n486 = Compound Arithmetic op=AND(w1051, w1043, w1036, invert w1037) -> (w1050:bool)
    }
    frame "ObjectValues" {
      w1057 = cluster{"a":i32, "b":string} {"a"=0, "b"=""} ("Cluster")
      w1055 = cluster{"a":i32, "b":string} {"a"=-123, "b"="Hello World"} ("Cluster")
      w1059 = "{\"a\":-123,\"b\":\"Hello World\"}"
      n487 = call "JSON Flatten.vi"("error in (no error)"=w1064, "Variant in"=w1055) -> ("error out"=w1065:errorcluster, "JSON out"=w1062:string)  [unwired: 8 in]
      n488 = call "JSON Unflatten.vi"("Variant Type"=w1057, "error in (no error)"=w1065, "JSON in"=w1062) -> ("error out"=w1063:errorcluster, "Exists?"=w1060:bool, "Variant out"=w1061:variant)  [unwired: 6 in]
      n489 = Variant To Data(error in=w1063, type=w1057, Variant=w1061) -> (data=w1053:cluster{"a":i32, "b":string}, error out=w1058:errorcluster)
      n490 = Variant To Flattened String(Variant=w1055) -> (data string=w1054:string)  [unwired: 1 out]
      n491 = Variant To Flattened String(Variant=w1053) -> (data string=w1052:string)  [unwired: 1 out]
      n492 = Equal?(x=w1054, y=w1052) -> (x = y?=w1056:bool)
      n493 = Equal?(x=w1059, y=w1062) -> (x = y?=w1068:bool)
      n494 = To Variant(anything=w1053) -> (Variant=w1066:variant)
      n495 = Compound Arithmetic op=AND(w1068, w1060, w1056, invert w1058) -> (w1067:bool)
    }
    frame "ObjectEmpty" {
      w1069 = cluster{"null":variant} {"null"=variant} ("Cluster")
      w1073 = cluster{variant} {variant} ("Cluster")
      w1076 = "{}"
      n496 = call "JSON Flatten.vi"("error in (no error)"=w1081, "Variant in"=w1073) -> ("error out"=w1082:errorcluster, "JSON out"=w1079:string)  [unwired: 8 in]
      n497 = call "JSON Unflatten.vi"("Variant Type"=w1069, "error in (no error)"=w1082, "JSON in"=w1079) -> ("error out"=w1080:errorcluster, "Exists?"=w1077:bool, "Variant out"=w1078:variant)  [unwired: 6 in]
      n498 = Variant To Data(error in=w1080, type=w1069, Variant=w1078) -> (data=w1071:cluster{"null":variant}, error out=w1075:errorcluster)
      n499 = Variant To Flattened String(Variant=w1073) -> (data string=w1072:string)  [unwired: 1 out]
      n500 = Variant To Flattened String(Variant=w1071) -> (data string=w1070:string)  [unwired: 1 out]
      n501 = Equal?(x=w1072, y=w1070) -> (x = y?=w1074:bool)
      n502 = Equal?(x=w1076, y=w1079) -> (x = y?=w1085:bool)
      n503 = To Variant(anything=w1071) -> (Variant=w1083:variant)
      n504 = Compound Arithmetic op=AND(w1085, w1077, w1074, invert w1075) -> (w1084:bool)
    }
    frame "ObjectWaveform" {
      w1092 = ext 1e-13  # EXT
      w1114 = waveform(dbl) {"t0"=timestamp(0 s since 1904-01-01), "dt"=1.0, "Y"=[]} ("Waveform")
      w1109 = waveform(dbl) {"t0"=timestamp(3681289404.123456 s since 1904-01-01), "dt"=0.5, "Y"=[1.1, 2.2, 3.3]} ("Waveform")
      n505 = Unbundle By Name(w1109) -> ("t0"=w1113:timestamp)
      n506 = Unbundle By Name(w1109) -> ("t0"=w1108:timestamp, "dt"=w1107:dbl, "Y"=w1106:dbl[])
      n507 = call "JSON Flatten.vi"("error in (no error)"=w1118, "Variant in"=w1109) -> ("error out"=w1119:errorcluster, "JSON out"=w1091:string)  [unwired: 8 in]
      n508 = call "JSON Timestamp to ISO8601.vi"("Local Date Time"=w1113) -> ("ISO 8601 Date Time"=w1112:string)  [unwired: 10 in]
      n509 = To Extended Precision Float(1:w1108) -> (0:w1105:ext)
      n510 = To Extended Precision Float(1:w1107) -> (0:w1104:ext)
      n511 = To Extended Precision Float(1:w1106) -> (0:w1103:ext[])
      n512 = call "JSON Unflatten.vi"("Variant Type"=w1114, "error in (no error)"=w1119, "JSON in"=w1091) -> ("error out"=w1117:errorcluster, "Exists?"=w1089:bool, "Variant out"=w1116:variant)  [unwired: 6 in]
      n513 = Format Into String(format string="{\"t0\":\"%s\",\"dt\":0.5,\"Y\":[1.1,2.2,3.3]}", w1112) -> (resulting string=w1110:string)  [unwired: 2 in, 1 out]
      n514 = Build Array (concatenate)(w1105, w1104, w1103) -> (w1090:ext[])
      n515 = Variant To Data(error in=w1117, type=w1114, Variant=w1116) -> (data=w1096:waveform(dbl), error out=w1115:errorcluster)
      n516 = Unbundle By Name(w1096) -> ("t0"=w1097:timestamp, "dt"=w1098:dbl, "Y"=w1099:dbl[])
      n517 = To Extended Precision Float(1:w1097) -> (0:w1100:ext)
      n518 = To Extended Precision Float(1:w1098) -> (0:w1101:ext)
      n519 = To Extended Precision Float(1:w1099) -> (0:w1102:ext[])
      n520 = Build Array (concatenate)(w1100, w1101, w1102) -> (w1088:ext[])
      n521 = Subtract(x=w1090, y=w1088) -> (x-y=w1095:ext[])
      n522 = Absolute Value(x=w1095) -> (abs(x)=w1094:ext[])
      n523 = Divide(x=w1094, y=w1088) -> (x/y=w1093:ext[])
      n524 = Less Or Equal?(x=w1093, y=w1092) -> (x <= y?=w1087:bool[])
      n525 = And Array Elements(Boolean array=w1087) -> (logical AND=w1086:bool)
      n526 = Equal?(x=w1110, y=w1091) -> (x = y?=w1122:bool)
      n527 = To Variant(anything=w1096) -> (Variant=w1120:variant)
      n528 = Compound Arithmetic op=AND(w1122, w1089, w1086, invert w1115) -> (w1121:bool)
    }
    frame "ObjectReorder" {
      w1131 = cluster{"b":string, "a":i32} {"b"="", "a"=0} ("Cluster")
      w1129 = cluster{"a":i32, "b":string} {"a"=-123, "b"="Hello World"} ("Cluster")
      w1133 = "{\"a\":-123,\"b\":\"Hello World\"}"
      n529 = call "JSON Flatten.vi"("error in (no error)"=w1138, "Variant in"=w1129) -> ("error out"=w1139:errorcluster, "JSON out"=w1136:string)  [unwired: 8 in]
      n530 = call "JSON Unflatten.vi"("Variant Type"=w1131, "error in (no error)"=w1139, "JSON in"=w1136) -> ("error out"=w1137:errorcluster, "Exists?"=w1134:bool, "Variant out"=w1135:variant)  [unwired: 6 in]
      n531 = Variant To Data(error in=w1137, type=w1131, Variant=w1135) -> (data=w1128:cluster{"b":string, "a":i32}, error out=w1132:errorcluster)
      n532 = Unbundle By Name(w1129) -> ("a"=w1127:i32, "b"=w1126:string)
      n533 = Unbundle By Name(w1128) -> ("b"=w1125:string, "a"=w1123:i32)
      n534 = Equal?(x=w1127, y=w1123) -> (x = y?=w1130:bool)
      n535 = Equal?(x=w1126, y=w1125) -> (x = y?=w1124:bool)
      n536 = Equal?(x=w1133, y=w1136) -> (x = y?=w1142:bool)
      n537 = To Variant(anything=w1128) -> (Variant=w1140:variant)
      n538 = Compound Arithmetic op=AND(w1142, w1134, w1130, w1124, invert w1132) -> (w1141:bool)
    }
  }
  "error out" <- w7
  "Passed?" <- w6
  "Result" <- w5
  "JSON in" <- w2
  "JSON out" <- w3
